vi "DriveExecute.vi"(8 "error in (no error)":errorcluster) -> (0 "error out":errorcluster)   [LabVIEW 2023]
doc: "Execute for Drie\n\nClosed control loop for drive\n\ninput: \n error in (cluster)\n\noutput:\n error out (cluster)"
uses:
  DriveGlobal.vi
  <vilib>/Rock Robotics/WPI/ThirdParty/JAS_Junk/TrajLib/Trajectory_Library.lvlib
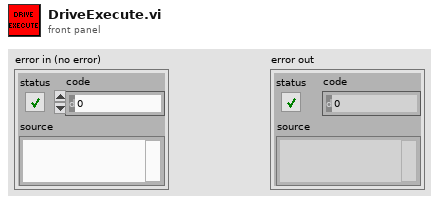
[diagram p1: front panel]
types:
  T1 = enum16{"Moving Average", "Low Pass 1st Order Butterworth", "Low Pass 2nd Order Butterworth", "High Pass 1st Order Butterworth", "High Pass 2nd Order Butterworth"}
  T2 = typedef "Trajectory_Library.lvlib/SWERVE_DRIVE_KINEMATICS.ctl" = cluster{"NumModules":i32, "InverseKinematics":T3, "ForwardKinematics":T3, "Modules":T4[], "PrevCoR":T4, "SavedModuleStates":T5[]}
  T3 = typedef "NI_Matrix.lvlib/RealMatrix.ctl" = dbl[][]
  T4 = typedef "Trajectory_Library.lvlib/TRANSLATION2D.ctl" = cluster{"X":dbl, "Y":dbl}
  T5 = typedef "Trajectory_Library.lvlib/SWERVE_DRIVE_MODULE_STATE.ctl" = cluster{"Speed":dbl, "Angle":T6}
  T6 = typedef "Trajectory_Library.lvlib/ROTATION2D.ctl" = cluster{"VALUE":dbl, "COS":dbl, "SIN":dbl}
  T7 = typedef "ADIS16470 Device Reference.ctl" = cluster{"DevStatus":errorcluster, "Hardware Config":T8, "Calibration Complete":refnum<notifier>, "Status Reference":refnum<data-value>, "Data Reference":refnum<data-value>, "Sychronous Process VI":T12, "Cmd FIFO":refnum<k33>, "Source":T13, "Data FIFO":refnum<k33>, "Calibration Time (ms)":u32, "Data Reference":refnum<data-value>}
  T8 = typedef "ADIS16470 Hardware Configuration.ctl" = cluster{"SPI Clock Rate (Hz)":dbl, "IMU SPI Mode (3)":T9, "IMU Reset Pin":T10, "IMU SPI Bus":T11, "IMU Data Ready Pin":T10, "Stall Config":cluster{"Pow2BytesPerRead":u8, "StallTicks":u16, "CsToSclkTicks":u8}}
  T9 = typedef "WPI_SPIMode.ctl" = enum16{"Mode 0 (Clk Idle Low,Sample on Leading)", "Mode 1 (Clk Idle Low,Sample on Trailing)", "Mode 2 (Clk Idle High,Sample on Leading)", "Mode 3 (Clk Idle High,Sample on Trailing)"}
  T10 = typedef "FPGA_DIOChannel.ctl" = enum8{"DIO 0", "DIO 1", "DIO 2", "DIO 3", "DIO 4", "DIO 5", "DIO 6", "DIO 7", "DIO 8", "DIO 9", "DIO MXP 0", "DIO MXP 1", "DIO MXP 2", "DIO MXP 3", "DIO MXP 4", "DIO MXP 5", "DIO MXP 6", "DIO MXP 7", "DIO MXP 8", "DIO MXP 9", "DIO MXP 10", "DIO MXP 11", "DIO MXP 12", "DIO MXP 13", "DIO MXP 14", "DIO MXP 15", "SPI Port CS1", "SPI Port CS2", "SPI Port CS3", "SPI Port MISO", "SPI Port MOSI", "Invalid"}
  T11 = typedef "spi_bus.ctl" = enum16{"SPI On-Board, CS0", "SPI On-Board, CS1", "SPI On-Board, CS2", "SPI On-Board, CS3", "SPI MXP", "Invalid"}
  T12 = typedef "ADIS16470 Process.ctl" = refnum<vi>
  T13 = typedef "FPGA_CounterEncoderSourceConvertionLVSourceType.ctl" = cluster{"DevStatus":errorcluster, "AnalogTriggerMode?":bool, "DigitalMode":cluster{"DIO Channel":T14}, "AnalogTriggerMode":cluster{"AnalogTriggerIndex":T15, "OutputType":T16}}
  T14 = typedef "FPGA_DIODigitalSourceChannel.ctl" = enum8{"DIO 0", "DIO 1", "DIO 2", "DIO 3", "DIO 4", "DIO 5", "DIO 6", "DIO 7", "DIO 8", "DIO 9", "DIO MXP 0", "DIO MXP 1", "DIO MXP 2", "DIO MXP 3", "DIO MXP 4", "DIO MXP 5", "DIO MXP 6", "DIO MXP 7", "DIO MXP 8", "DIO MXP 9", "DIO MXP 10", "DIO MXP 11", "DIO MXP 12", "DIO MXP 13", "DIO MXP 14", "DIO MXP 15", "SPI Port CS1", "SPI Port CS2", "SPI Port CS3", "SPI Port MISO", "SPI Port MOSI", "Disabled"}
  T15 = typedef "FPGA_AnalogTriggerIndex.ctl" = enum8{"Trig 0", "Trig 1", "Trig 2", "Trig 3", "Trig 4", "Trig 5", "Trig 6", "Trig 7", "Invalid"}
  T16 = typedef "FPGA_AnalogTriggerOutType.ctl" = enum16{"InWindow", "TriggerState", "Rising", "Falling"}
  T17 = typedef "ADIS16470 Data.ctl" = cluster{"XAngle":dbl, "YAngle":dbl, "ZAngle":dbl}
  T18 = typedef "ADIS16470 Status.ctl" = cluster{"Calibrated?":bool, "IMU Detected?":bool}
  T19 = typedef "Trajectory_Library.lvlib/CHASSIS_SPEEDS.ctl" = cluster{"vX":dbl, "vY":dbl, "vOmega":dbl}
  T20 = typedef "Trajectory_Library.lvlib/SWERVE_DRIVE_MODULE_POSITION.ctl" = cluster{"Distance":dbl, "Angle":T6, "P":bool}
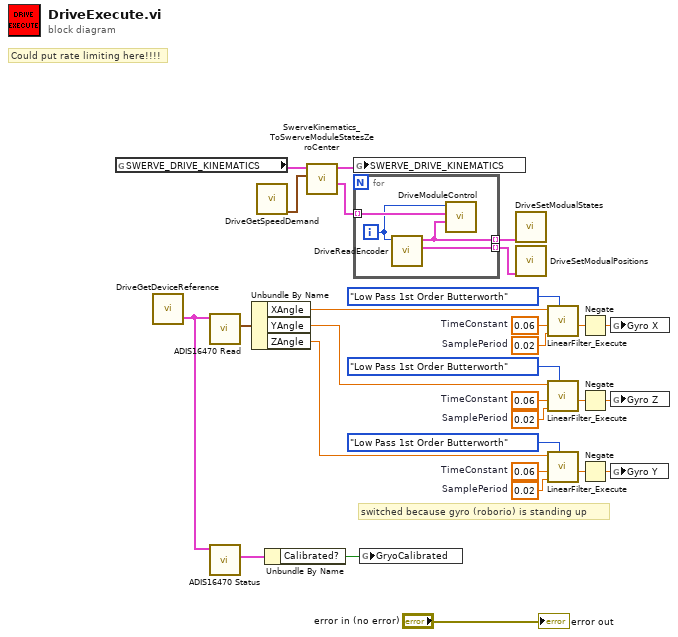
[diagram p0: block diagram]
diagram:
  w14 = 0.02  # SamplePeriod
  w13 = 0.06  # TimeConstant
  w19 = 0.02  # SamplePeriod
  w18 = 0.06  # TimeConstant
  w24 = 0.02  # SamplePeriod
  w23 = 0.06  # TimeConstant
  # "Could put rate limiting here!!!!"
  # "switched because gyro (roborio) is standing up"
  n1 = global read "DriveGlobal.vi" "SWERVE_DRIVE_KINEMATICS"() -> (w8:T2)
  n2 = call "DriveGetDeviceReference.vi"() -> ("Gryo"=w25:T7)  [unwired: 11 in]
  n3 = call <vilib>:"ADIS16470 Read.vi"("ADIS16470DevRef"=w25) -> ("ADIS16470 Value"=w28:T17)  [unwired: 7 in, 3 out]
  n4 = call <vilib>:"ADIS16470 Status.vi"("ADIS16470DevRef"=w25) -> ("ADIS16470 Status"=w27:T18)  [unwired: 8 in, 2 out]
  n5 = Unbundle By Name(w28) -> ("XAngle"=w9:dbl, "YAngle"=w15:dbl, "ZAngle"=w21:dbl)
  n6 = call "DriveGetSpeedDemand.vi"() -> ("ChassisSpeedDemand"=w7:T19)  [unwired: 8 in, 3 out]
  n7 = Unbundle By Name(w27) -> ("Calibrated?"=w26:bool)
  n8 = call <vilib>:"SwerveKinematics_ToSwerveModuleStatesZeroCenter.vi"("ChassisSpeeds"=w7, "in SWERVE_DRIVE_KINEMATICS"=w8) -> ("ModuleStates"=w3:T5[], "out SWERVE_DRIVE_KINEMATICS"=w6:T2)  [unwired: 8 in]
  n9 = global write "DriveGlobal.vi" "SWERVE_DRIVE_KINEMATICS"(w6) -> ()
  n10 = for {
    tunnel: w3 -> [w33] mode=indexing
    tunnel: [w31] -> w2 mode=indexing
    tunnel: [w30] -> w1 mode=indexing
    i -> [w32]
    n11 = call "DriveReadEncoder.vi"("ModualNamePrefix"=w32) -> ("SWERVE_DRIVE_MODULE_POSITION"=w31:T20, "SWERVE_DRIVE_MODULE_STATE"=w30:T5)  [unwired: 8 in, 1 out]
    n12 = call "DriveModuleControl.vi"("Actual State"=w30, "Desired State"=w33, "ModualNamePrefix"=w32) -> ()  [unwired: 8 in, 1 out]
  }
  n13 = global write "DriveGlobal.vi" "GryoCalibrated"(w26) -> ()
  n14 = call "DriveSetModualStates.vi"("Swerve__Drive_Modual_States"=w1) -> ()  [unwired: 11 in]
  n15 = call "DriveSetModualPositions.vi"("Swerve_Drive_Modual_Position"=w2) -> ()  [unwired: 11 in]
  n16 = call <vilib>:"LinearFilter_Execute.vi"("Filter Type"=T1."Low Pass 1st Order Butterworth", "SamplePeriod"=w14, "TimeConstant"=w13, "Input"=w9) -> ("Output"=w11:dbl)  [unwired: 6 in, 1 out]
  n17 = call <vilib>:"LinearFilter_Execute.vi"("Filter Type"=T1."Low Pass 1st Order Butterworth", "SamplePeriod"=w19, "TimeConstant"=w18, "Input"=w15) -> ("Output"=w16:dbl)  [unwired: 6 in, 1 out]
  n18 = call <vilib>:"LinearFilter_Execute.vi"("Filter Type"=T1."Low Pass 1st Order Butterworth", "SamplePeriod"=w24, "TimeConstant"=w23, "Input"=w21) -> ("Output"=w20:dbl)  [unwired: 6 in, 1 out]
  n19 = Negate(x=w11) -> (-x=w10:dbl)
  n20 = Negate(x=w16) -> (-x=w5:dbl)
  n21 = Negate(x=w20) -> (-x=w4:dbl)
  n22 = global write "DriveGlobal.vi" "Gyro X"(w10) -> ()
  n23 = global write "DriveGlobal.vi" "Gyro Z"(w5) -> ()
  n24 = global write "DriveGlobal.vi" "Gyro Y"(w4) -> ()
  "error out" <- "error in (no error)"
